vi "Send Command and Wait for Response.vi"(8 "error in":errorcluster, 9 "timeout":i32=2000, 10 "cmd queue":refnum<queue>, 11 "CMD in":refnum<class "Command.lvclass">) -> (0 "error out":errorcluster, 2 "cmd good?":bool, 3 "CMD out":refnum<class "Command.lvclass">)   [LabVIEW 2016, in "Command.lvclass"]
doc: "Use this VI to send a command when a reply is expected. If no reply is necessary, simply write the command to the appropriate command queue. This VI populates the reply queue with a freshly created queue. After the message is sent, the VI will wait the amount of time supplied in the timeout before returning. To wait indefinitely, set the timeout to -1."
uses:
  Command.lvclass
  Command.lvclass/Command.ctl
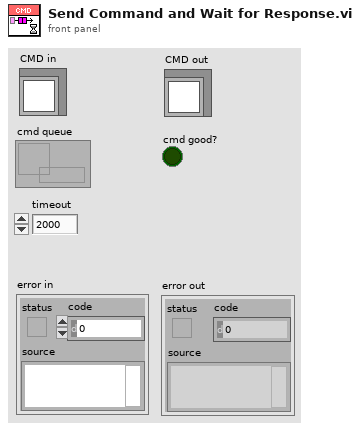
[diagram p1: front panel]
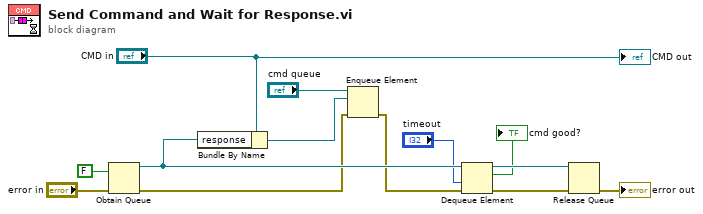
[diagram p0: block diagram]
diagram:
  n1 = Obtain Queue(element data type=FALSE, error in (no error)="error in") -> (queue out=w9:refnum<queue>, error out=w4:errorcluster)  [unwired: 3 in, 1 out]
  n2 = Bundle By Name(cluster="CMD in", "response"=w9) -> (w10:refnum<class "Command.lvclass">)
  n3 = Enqueue Element(queue="cmd queue", element=w10, error in (no error)=w4) -> (error out=w3:errorcluster)  [unwired: 1 in, 2 out]
  n4 = Dequeue Element(queue=w9, timeout in ms (-1)="timeout", error in (no error)=w3) -> (queue out=w8:refnum<queue>, element=→"cmd good?":bool, error out=w7:errorcluster)  [unwired: 1 out]
  n5 = Release Queue(queue=w8, error in (no error)=w7) -> (error out=→"error out":errorcluster)  [unwired: 1 in, 2 out]
  "CMD out" <- "CMD in"
